vi "Edited_struc.vi"() -> ()   [LabVIEW 2021]
uses:
  <vilib>/numeric/Random Number (Range) I64.vi
  <vilib>/numeric/sub_Random U32.vi
panel:
  in  "Boolean":bool
  out "Waveform Graph":i32[](graph)
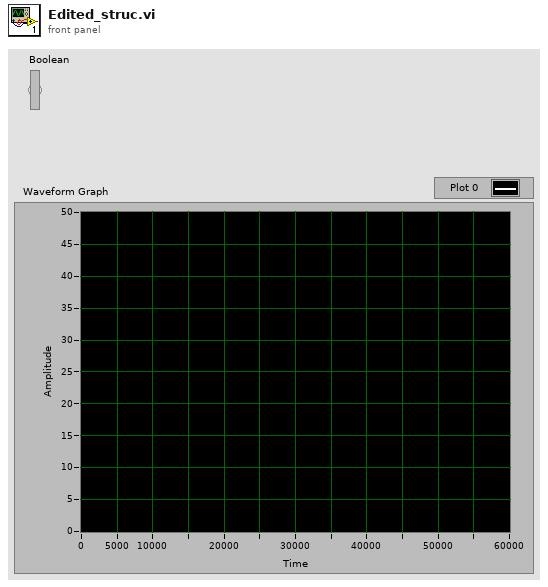
[diagram p1: front panel]
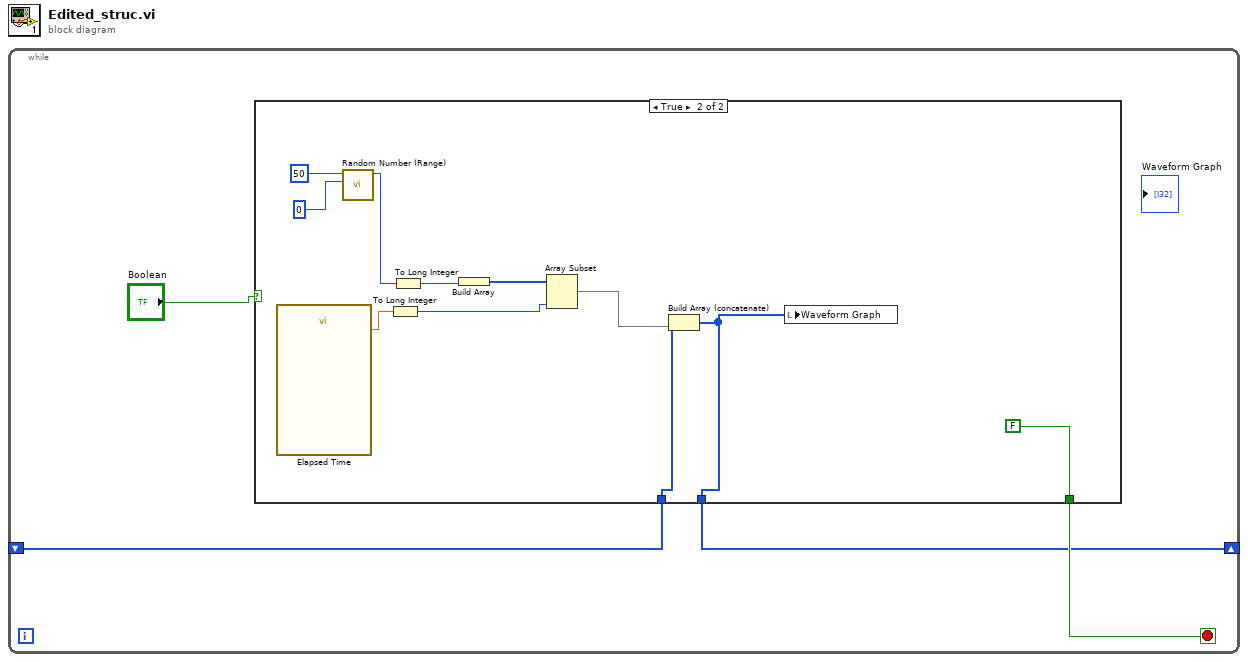
[diagram p0: block diagram]
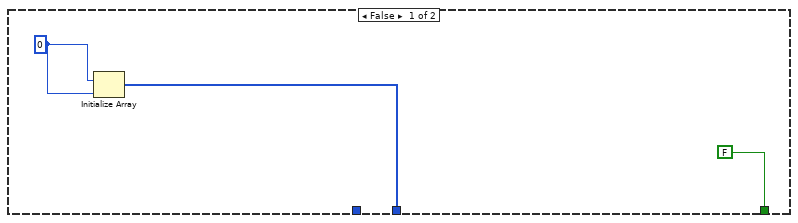
[diagram p2: hidden frame]
diagram:
  n1 = while {
    shift-right: [w1] -> _
    shift-left: _ -> [w4]
    stop <- w3 stop-if-true
    n2 = case shown="True" "Boolean" {
      tunnel: [w6 w8] -> w1
      tunnel: w4 -> [_ w10]
      tunnel: [FALSE FALSE] -> w3
      frame False {
        w7 = 0
        n3 = Initialize Array(w7, w7) -> (w6:i32[])
      }
      frame True {
        n4 = call "Elapsed Time"() -> ("Elapsed Time (s)"=w15:dbl)  [unwired: 12 in, 7 out]
        n5 = call-poly <vilib>:"Random Number (Range).vi"("lower bound (-100)"=0, "upper bound (100)"=50) -> ("number"=w16:i64)  [unwired: 9 in]
        n6 = To Long Integer(number=w15) -> (32bit integer=w14:i32)
        n7 = To Long Integer(number=w16) -> (32bit integer=w13:i32)
        n8 = Build Array(w13) -> (w12:i32[])
        n9 = Array Subset(array=w12, length=w14) -> (w11:i32[])  [unwired: 1 in]
        n10 = Build Array (concatenate)(w10, w11) -> (w8:i32[])
        n11 = local write "Waveform Graph"(w8) -> ()
      }
    }
  }
